vi "sequence.vi"(8 "error in (no error)":errorcluster, 11 "ScriptEventList in":refnum<class "ScriptEventList.lvclass">) -> (0 "error out":errorcluster, 1 "allStrings":string[][](array[string]), 2 "sequencedArray":refnum<class "ScriptEvent.lvclass">[](array[class]), 3 "ScriptEventList out":refnum<class "ScriptEventList.lvclass">)   [LabVIEW 2011, in "Tools.lvlib" / "Scripting.lvlib" / "ScriptEventList.lvclass"]
uses:
  ScriptEventList.lvclass
  ScriptEvent.lvclass
  ScriptEventList.lvclass/ScriptEventList.ctl
  DatabaseHelpers/Database Objects/Channel/Channel.lvclass
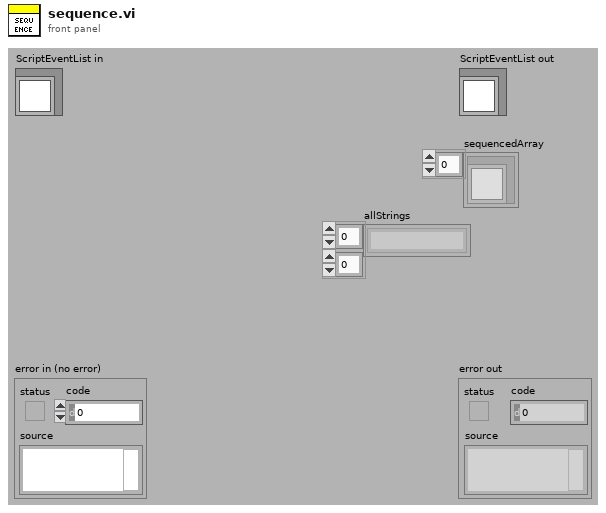
[diagram p1: front panel]
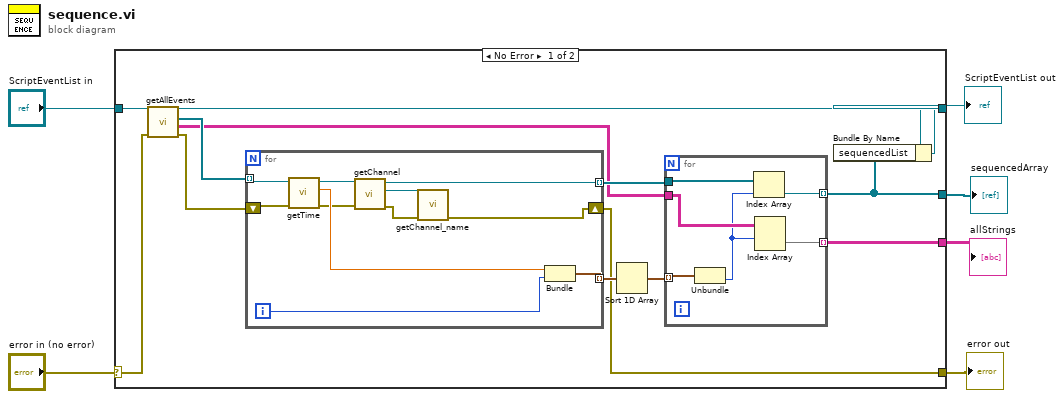
[diagram p0: block diagram]
diagram:
  n1 = case shown="No Error" "error in (no error)" {
    selector: "error in (no error)" -> [w18 w38]
    tunnel: [w12 w38] -> w5
    tunnel: [w10 w37] -> w3
    tunnel: "ScriptEventList in" -> [w19 w37]
    tunnel: [w9 _] -> w2
    tunnel: [w7 _] -> w1
    frame No Error {
      n2 = call "getAllEvents.vi"("error in (no error)"=w18, "ScriptEventList in"=w19) -> ("error out"=w16:errorcluster, "allStrings"=w8:string[][], "allScriptEvents"=w17:refnum<class "ScriptEvent.lvclass">[], "ScriptEventList out"=w11:refnum<class "ScriptEventList.lvclass">)  [unwired: 6 in]
      n3 = for {
        tunnel: w17 -> [w36] mode=indexing
        shift-right: [w30] -> w12
        shift-left: w16 -> [w35]
        tunnel: [w31] -> w15 mode=indexing
        tunnel: [w29] -> w13 mode=indexing
        i -> [w28]
        n4 = call "getTime.vi"("error in (no error)"=w35, "ScriptEvent.lvclass in"=w36) -> ("error out"=w26:errorcluster, "time"=w32:dbl, "ScriptEvent.lvclass out"=w27:refnum<class "ScriptEvent.lvclass">)  [unwired: 7 in]
        n5 = call-dynamic "getChannel.vi"("error in (no error)"=w26, "ScriptEvent.lvclass in"=w27) -> ("error out"=w33:errorcluster, "Channel.lvclass"=w34:refnum<class "Channel.lvclass">, "ScriptEvent.lvclass out"=w29:refnum<class "ScriptEvent.lvclass">)  [unwired: 7 in]
        n6 = call "getChannel_name.vi"("error in (no error)"=w33, "Channel.lvclass in"=w34) -> ("error out"=w30:errorcluster)  [unwired: 7 in, 2 out]
        n7 = Bundle("time"=w32, w28) -> (w31:cluster{"time":dbl, i32})  [unwired: 1 in]
      }
      n8 = Sort 1D Array(array=w15) -> (sorted array=w14:cluster{"time":dbl, i32}[])
      n9 = for {
        tunnel: w14 -> [w24] mode=indexing
        tunnel: w13 -> [w25]
        tunnel: [w23] -> w9 mode=indexing
        tunnel: w8 -> [w22]
        tunnel: [w21] -> w7 mode=indexing
        n10 = Unbundle(w24) -> (w20:i32)  [unwired: 1 out]
        n11 = Index Array(array=w25, index=w20) -> (element=w23:refnum<class "ScriptEvent.lvclass">)
        n12 = Index Array(array=w22, index (row)=w20) -> (element=w21:string[])  [unwired: 1 in]
      }
      n13 = Bundle By Name(cluster=w11, "sequencedList"=w9) -> (w10:refnum<class "ScriptEventList.lvclass">)
    }
    frame Error {
    }
  }
  "error out" <- w5
  "ScriptEventList out" <- w3
  "sequencedArray" <- w2
  "allStrings" <- w1
